vi "begin5RobotsKeeperGame.vi"(8 "error in (no error)":errorcluster, 9 "Game in":refnum<class "Game.lvclass">, 10 "command_interpreted":T1, 11 "5RobotsKeeperGame in":refnum<class "5RobotsKeeperGame.lvclass">) -> (0 "error out":errorcluster, 2 "begin?":bool, 3 "5RobotsKeeperGame out":refnum<class "5RobotsKeeperGame.lvclass">)   [LabVIEW 2021, in "5RobotsKeeperGame.lvclass"]
uses:
  5RobotsKeeperGame.lvclass
  Game_class/Game.lvclass
  Referee_class/command_interpreted.ctl
  Utilities_class/Utilities.lvclass
  Game_class/Game.lvclass/Game.ctl
  Team_class/Team.lvclass/Team.ctl
  Object_class/Object.lvclass/Object.ctl
  Game_class/Read AllyRef.vi
  Game_class/Read OffensiveTeam.vi
  Game_class/Read BallRef.vi
  Game_class/Read Utilities.lvclass.vi
  Object_class/Read x.vi
  Object_class/Read y.vi
  Team_class/Read RobotRef.vi
  Ball_class/Ball.lvclass
  D:/RoboIme/horie/SSL_AI/Object_class/Object.lvclass
  Ally_class/Ally.lvclass
  D:/RoboIme/horie/SSL_AI/Team_class/Team.lvclass
  Robot_class/Robot.lvclass
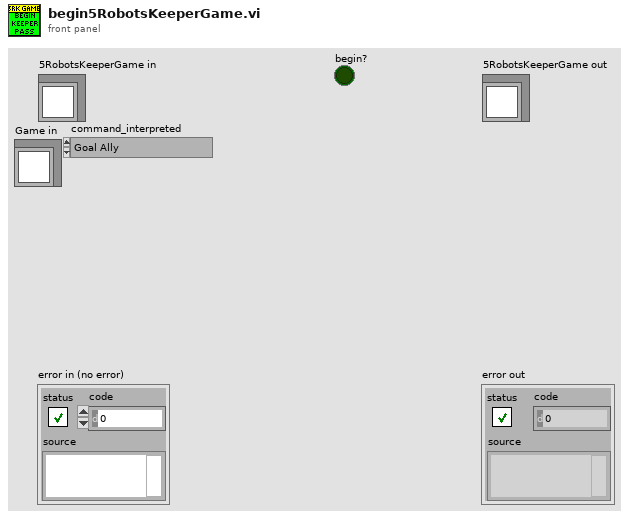
[diagram p1: front panel]
types:
  T1 = typedef "command_interpreted.ctl" = enum16{"Goal Ally", "Goal Enemy", "Ball Placement Enemy", "Ball Placement Ally", "Normal Half Time", "Extra Time  Break", "Extra Half Time", "None", "Post Game", "PKA Normal Start", "Prepare Kickoff Ally", "PKE Normal Start", "Prepare Kickoff Enemy", "Force Start", "Halt", "Timeout", "Prepare Penalty Ally", "Prepare Penalty Enemy", "PPA NormalStart", "PPE Normal Start", "Indirect Free Ally", "Direct Free Enemy", "Direct Free Ally", "Indirect Free Enemy", "Stop"}
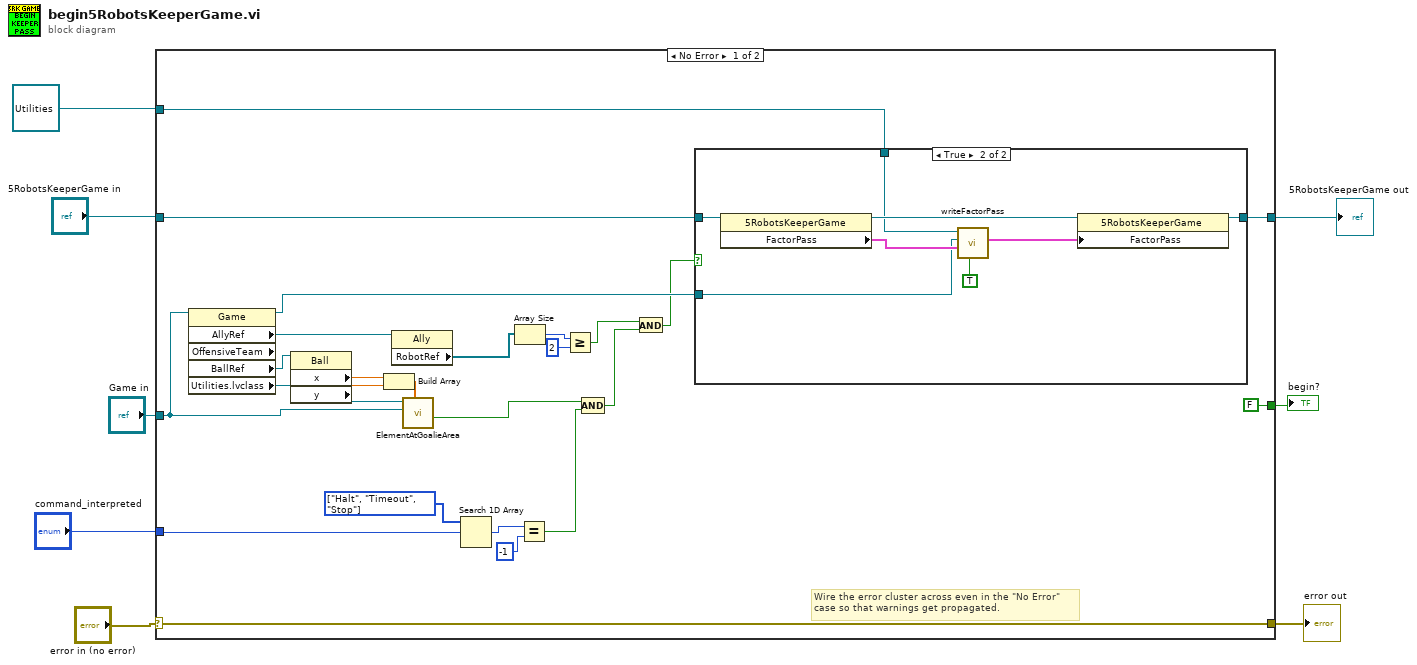
[diagram p0: block diagram]
diagram:
  n1 = case shown="No Error" "error in (no error)" {
    selector: "error in (no error)" -> [w33 w44]
    tunnel: [w33 w44] -> w8
    tunnel: [w19 w43] -> w5
    tunnel: "5RobotsKeeperGame in" -> [w20 w43]
    tunnel: "Game in" -> [w32 _]
    tunnel: [FALSE _] -> w4
    tunnel: "command_interpreted" -> [w23 _]
    tunnel: refnum<class "Utilities.lvclass"> refnum ("Utilities in") -> [w18 _]
    frame No Error {
      w26 = T1[] [enum."Halt", enum."Timeout", enum."Stop"] items=["Goal Ally", "Goal Enemy", "Ball Placement Enemy", "Ball Placement Ally", "Normal Half Time", "Extra Time  Break", "Extra Half Time", "None", "Post Game", "PKA Normal Start", "Prepare Kickoff Ally", "PKE Normal Start", "Prepare Kickoff Enemy", "Force Start", "Halt", "Timeout", "Prepare Penalty Ally", "Prepare Penalty Enemy", "PPA NormalStart", "PPE Normal Start", "Indirect Free Ally", "Direct Free Enemy", "Direct Free Ally", "Indirect Free Enemy", "Stop"] ("Array")
      # "Wire the error cluster across even in the \"No Error\"\ncase so that warnings get propagated."
      n2 = property class="Game" props=["AllyRef", "OffensiveTeam", "BallRef", "Utilities.lvclass"](reference=w32) -> (reference out=w17:refnum<class "Game.lvclass">, "AllyRef"=w13:refnum<class "Ally.lvclass">, "BallRef"=w31:refnum<class "Ball.lvclass">, "Utilities.lvclass"=w21:refnum<class "Utilities.lvclass">)  [unwired: 1 in, 2 out]
      n3 = property class="Ball"(reference=w31) -> ("x"=w30:dbl, "y"=w29:dbl)  [unwired: 1 in, 2 out]
      n4 = Build Array(w30, w29) -> (w28:dbl[])
      n5 = property class="Ally"(reference=w13) -> ("RobotRef"=w12:refnum<class "Robot.lvclass">[])  [unwired: 1 in, 2 out]
      n6 = call "ElementAtGoalieArea.vi"("Elemento pos."=w28, "Game"=w32, "Utilities in"=w21) -> ("Element at our goalkeeper area ?"=w27:bool)  [unwired: 4 in, 4 out]
      n7 = Search 1D Array(1D array=w26, element=w23) -> (index of element=w25:i32)  [unwired: 1 in]
      n8 = Array Size(array=w12) -> (size(s)=w16:i32)
      n9 = Equal?(x=w25, y=-1) -> (x = y?=w22:bool)
      n10 = Greater Or Equal?(x=w16, y=2) -> (x >= y?=w11:bool)
      n11 = Compound Arithmetic op=AND(w27, w22) -> (w10:bool)
      n12 = And(x=w11, y=w10) -> (x .and. y?=w14:bool)
      n13 = case shown="True" w14 {
        tunnel: w20 -> [w34 w42]
        tunnel: [w34 w40] -> w19
        tunnel: w18 -> [_ w38]
        tunnel: w17 -> [_ w37]
        frame False {
        }
        frame True {
          n14 = property class="5RobotsKeeperGame"(reference=w42) -> (reference out=w41:refnum<class "5RobotsKeeperGame.lvclass">, "FactorPass"=w39:cluster{"id":dbl[], "value":dbl[]})  [unwired: 1 in, 1 out]
          n15 = call "writeFactorPass.vi"("Pass?"=TRUE, "FactorPass in"=w39, "Game in"=w37, "Utilities in"=w38) -> ("FactorPass out"=w35:cluster{"id":dbl[], "value":dbl[]})  [unwired: 3 in, 4 out]
          n16 = property class="5RobotsKeeperGame"(reference=w41, "FactorPass"=w35) -> (reference out=w40:refnum<class "5RobotsKeeperGame.lvclass">)  [unwired: 1 in, 1 out]
        }
      }
    }
    frame Error {
    }
  }
  "error out" <- w8
  "5RobotsKeeperGame out" <- w5
  "begin?" <- w4
